vi "Build Type String.vi"(11 "Package Build in":refnum<class "Package Build.lvclass">) -> (2 "Build Type":string)   [LabVIEW 2020, in "Builder Tools.lvlib" / "Package Build.lvclass"]
uses:
  Package Build.lvclass
  Package Build.lvclass/Package Build.ctl
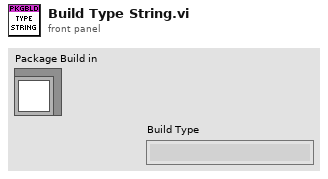
[diagram p1: front panel]
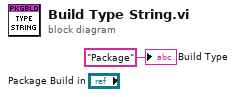
[diagram p0: block diagram]
diagram:
  "Build Type" <- "Package" ("Build Type")
